vi "Actuators Wait for Move.vi"(0 "Notifier Name":string, 2 "Timeout (ms)":i32=10000, 5 "Channel":i32, 11 "Error In":errorcluster) -> (4 "Notifier Name Out":string, 6 "Channel Out":i32, 15 "Error Out":errorcluster)   [LabVIEW 2020]
uses:
  Actuators Controls/Actuators Note Type.ctl
  Actuators Controls/Actuators Actions.ctl
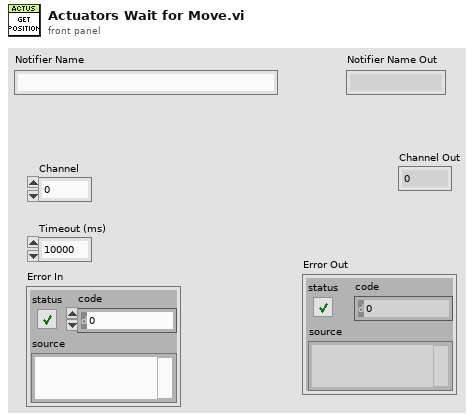
[diagram p1: front panel]
types:
  T1 = typedef "Actuators Note Type.ctl" = cluster{"Actions":T2, "Cmd Received ":bool, "Setpoint":dbl[], "Position":dbl[], "Channel":i32[], "Jog Step":dbl[], "Velocity":dbl[], "Acceleration":dbl[], "Status Bits":u32[], "Moving":bool[]}
  T2 = typedef "Actuators Actions.ctl" = enum16{"Nothing", "Get Position", "Get Acceleration", "Get Velocity", "Get Jog Step", "Set Acceleration", "Set Velocity", "Set Jog Step", "Move Absolute", "Move Relative", "Jog Forward", "Jog Reverse", "Set Moving", "Halt", "Quit"}
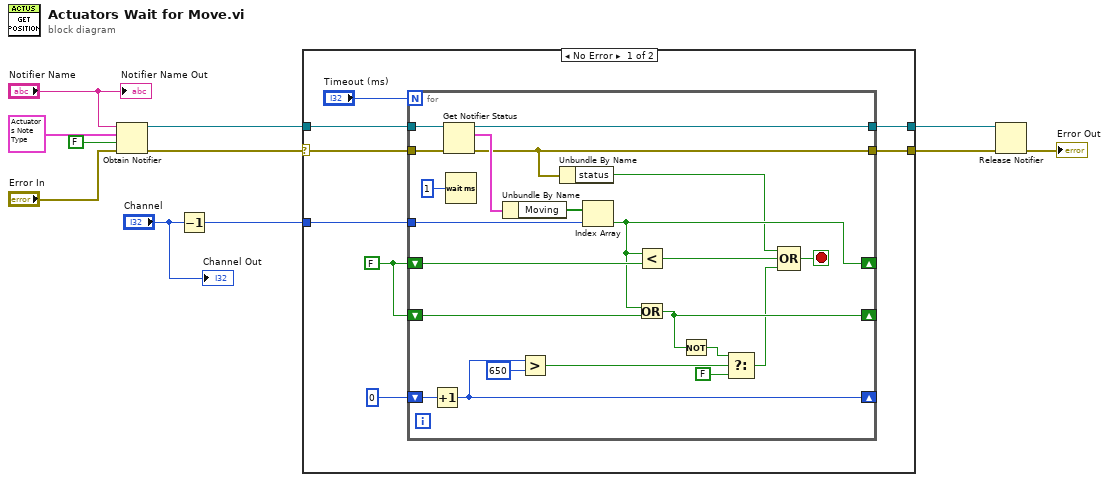
[diagram p0: block diagram]
diagram:
  n1 = Obtain Notifier(name (unnamed)="Notifier Name", notification data type=T1 {"Actions"=enum."Nothing", "Cmd Received "=FALSE, "Setpoint"=[], "Position"=[], "Channel"=[], "Jog Step"=[], "Velocity"=[], "Acceleration"=[], "Status Bits"=[], "Moving"=[]} ("Actuators Note"), create if not found? (T)=FALSE, error in (no error)="Error In") -> (notifier out=w7:refnum<notifier>, error out=w10:errorcluster)  [unwired: 1 out]
  n2 = Decrement(x="Channel") -> (x-1=w1:i32)
  n3 = case shown="No Error" w10 {
    selector: w10 -> [w18 w42]
    tunnel: w7 -> [w19 w43]
    tunnel: [w17 w43] -> w6
    tunnel: [w15 w42] -> w5
    tunnel: w1 -> [w16 _]
    frame No Error {
      w13 = FALSE
      n4 = for {
        N: "Timeout (ms)" -> [_]
        shift-right: [w31] -> _
        shift-left: w13 -> [w41]
        tunnel: w19 -> [w38]
        tunnel: w18 -> [w37]
        tunnel: [w36] -> w17
        tunnel: w16 -> [w34]
        tunnel: [w33] -> w15
        shift-right: [w26] -> _
        shift-left: w13 -> [w32]
        shift-right: [w29] -> _
        shift-left: u16 0 -> [w30]
        stop <- w20 stop-if-true
        n5 = Increment(x=w30) -> (x+1=w29:u16)
        n6 = Get Notifier Status(notifier=w38, error in (no error)=w37) -> (notifier out=w36:refnum<notifier>, current notification=w39:T1, error out=w33:errorcluster)  [unwired: 2 out]
        n7 = Wait (ms)(milliseconds to wait=u32 1) -> ()  [unwired: 1 out]
        n8 = Unbundle By Name(w39) -> ("Moving"=w35:bool[])
        n9 = Greater?(x=w29, y=u16 650) -> (0:w27:bool)
        n10 = Unbundle By Name(w33) -> ("status"=w21:bool)
        n11 = Index Array(array=w35, index=w34) -> (element=w31:bool)
        n12 = Less?(x=w31, y=w41) -> (x < y?=w23:bool)
        n13 = Or(x=w31, y=w32) -> (x .or. y?=w26:bool)
        n14 = Not(x=w26) -> (.not. x?=w25:bool)
        n15 = Select(t=w25, s=w27, f=FALSE) -> (s? t:f=w22:bool)
        n16 = Compound Arithmetic op=OR(w21, w23, w22) -> (w20:bool)
      }
    }
    frame Error {
    }
  }
  n17 = Release Notifier(notifier=w6, error in (no error)=w5) -> (error out=→"Error Out":errorcluster)  [unwired: 1 in, 2 out]
  "Notifier Name Out" <- "Notifier Name"
  "Channel Out" <- "Channel"
